vi "PointerToArray.vi"(8 "error in (no error)":errorcluster, 9 "Pointer In":u64, 10 "Array in":u8[](array[numeric])) -> (0 "error out":errorcluster, 2 "Array out":u8[](array[numeric]))   [LabVIEW 2019]
doc: "Pointer To Array\n\nOutput:\n U8[] Array out \n\nInput:\n U8[] Array in\n U64 Pointer in\n\nPopulates an array from its pointer."
uses:
  <vilib>/Utility/importsl/GetValueByPointer/datatype.ctl
  <vilib>/Utility/importsl/GetValueByPointer/GetValueByPointer.xnode
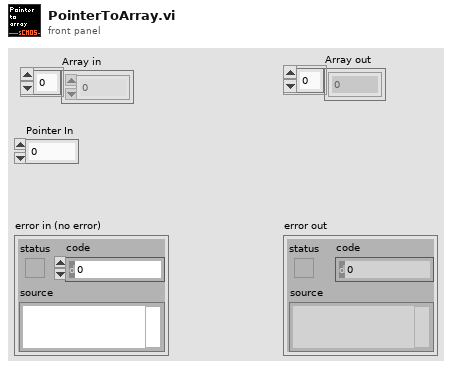
[diagram p1: front panel]
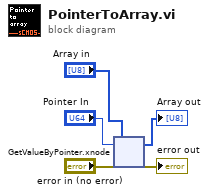
[diagram p0: block diagram]
diagram:
  n1 = xnode "GetValueByPointer.xnode"("Pointer"="Pointer In", "InputType"="Array in", "ErrorIn"="error in (no error)") -> ("Output"=→"Array out":u8[], "ErrorOut"=→"error out":errorcluster)  [unwired: 1 in]
